vi "SwerveShortestTurnAlg.vi"(8 "SwerveMotorsFlipped?":bool, 9 "SwerveSpeed":dbl, 10 "AngleSetpoint":dbl, 11 "AngleEncoder":dbl) -> (2 "FlipSwerveMotors":bool, 3 "PIDInput":dbl)   [LabVIEW 2018]
uses:
  SwerveGlobals.vi
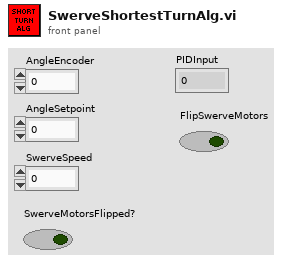
[diagram p1: front panel]
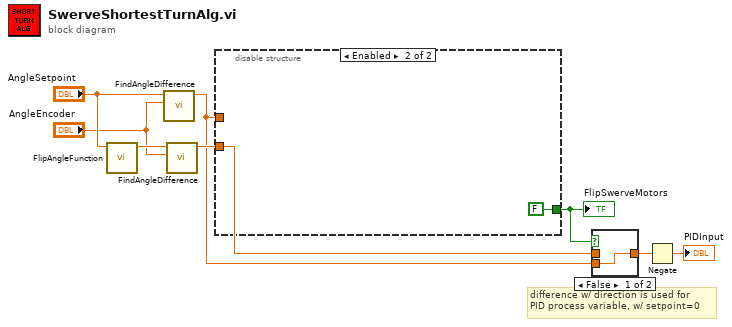
[diagram p0: block diagram]
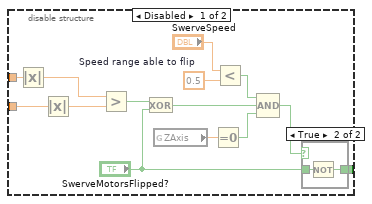
[diagram p2: hidden frame]
diagram:
  # "difference w/ direction is used for\nPID process variable, w/ setpoint=0"
  n1 = call "FlipAngleFunction.vi"("AngleInput"="AngleSetpoint") -> ("AngleFlipped"=w4:dbl)  [unwired: 10 in]
  n2 = call "FindAngleDifference.vi"("AngleEncoder"="AngleEncoder", "AngleSetpoint"="AngleSetpoint") -> ("Distance/DirectionOfTurn"=w2:dbl)  [unwired: 9 in]
  n3 = call "FindAngleDifference.vi"("AngleEncoder"="AngleEncoder", "AngleSetpoint"=w4) -> ("Distance/DirectionOfTurn"=w5:dbl)  [unwired: 9 in]
  n4 = disable-structure shown="Enabled" {
    disable-tunnel: [w13 FALSE ("FlipSwerveMotors")] -> w8
    disable-tunnel: w2 -> [w12 _]
    disable-tunnel: w5 -> [w9 _]
    frame Disabled {
      w22 = 0.5  # Speed range able to flip
      n5 = Absolute Value(x=w12) -> (abs(x)=w11:dbl)
      n6 = Absolute Value(x=w9) -> (abs(x)=w10:dbl)
      n7 = Greater?(x=w11, y=w10) -> (0:w19:bool)
      n8 = Exclusive Or(1:"SwerveMotorsFlipped?", 2:w19) -> (0:w16:bool)
      n9 = global read "SwerveGlobals.vi" "ZAxis"() -> (w21:dbl)
      n10 = Equal To 0?(x=w21) -> (x = 0?=w15:bool)
      n11 = Less?(x="SwerveSpeed", y=w22) -> (x < y?=w17:bool)
      n12 = Compound Arithmetic op=AND(w17, w16, w15) -> (w14:bool)
      n13 = case shown="True" w14 {
        tunnel: "SwerveMotorsFlipped?" -> [w23 w25]
        tunnel: [w23 w24] -> w13
        frame False {
        }
        frame True {
          n14 = Not(x=w25) -> (.not. x?=w24:bool)
        }
      }
    }
    frame Enabled {
    }
  }
  "FlipSwerveMotors" <- w8
  n15 = case shown="False" w8 {
    tunnel: w2 -> [w27 _]
    tunnel: w5 -> [_ w28]
    tunnel: [w27 w28] -> w7
    frame False {
    }
    frame True {
    }
  }
  n16 = Negate(x=w7) -> (-x=→"PIDInput":dbl)
